vi "LakeShore 336 Curve Manager.vi"() -> ()   [LabVIEW 2021]
doc: "VI to manage calibration curves in Lakeshore model 370 AC resistance Bridge. It will upload, download and display or delete curves. It will always delete a curve before uploading so the input setup may have to be reset after an upload.\nScott Hannahs, <sth@magnet.fsu.edu> NHMFL-FSU, May 2003"
uses:
  Misc Extras/Manufacturer Drivers/LakeShore/Lake Shore Cryotronics 336/Public/Utility/Data Format.ctl
  Sub Controls/ThermListIndex.ctl
  Misc Extras/Manufacturer Drivers/LakeShore/Lake Shore Cryotronics 336/Lake Shore 336.lvlib
panel:
  in  "Done2":bool
  out "XY Graph":cluster{dbl[], dbl[]}(graph)
  out "Curve #":u32[](array[numeric])
  in  "ThermListIndex":T1 max=40 step=20
  in  "stop":bool
  in  "Replace":bool[](array[boolean])=[FALSE, FALSE, FALSE, FALSE, FALSE, FALSE, FALSE, FALSE, FALSE, FALSE, FALSE, FALSE, FALSE, FALSE, FALSE, FALSE, FALSE, FALSE, FALSE, FALSE]
  in  "View":bool[](array[boolean])=[FALSE, FALSE, FALSE, FALSE, FALSE, FALSE, FALSE, FALSE, FALSE, FALSE, FALSE, FALSE, FALSE, FALSE, FALSE, FALSE, FALSE, FALSE, FALSE, FALSE]
  in  "Delete":bool[](array[boolean])=[FALSE, FALSE, FALSE, FALSE, FALSE, FALSE, FALSE, FALSE, FALSE, FALSE, FALSE, FALSE, FALSE, FALSE, FALSE, FALSE, FALSE, FALSE, FALSE, FALSE]
  out "Thermometer List":T3(array[cluster]) {"Temp. Coef" items=["????", "Negative", "Positive"]; "Setpoint Limit" format="%.4f"; "Data Format" items=["mV/K"=1, "V/K"=2, "Ω/K"=3, "Log Ω/K"=4]}
  in  "VISA session":refnum<visa-resource-name>
  out "Model":string="LakeShore Model 370"
  out "Info":string="S/N #000000, Software Date: 20030622"
  # "Name"
  # "Serial #"
  # "Data Format"
  # "Setpoint Limit"
  # "Temp. Coef"
  # "`"
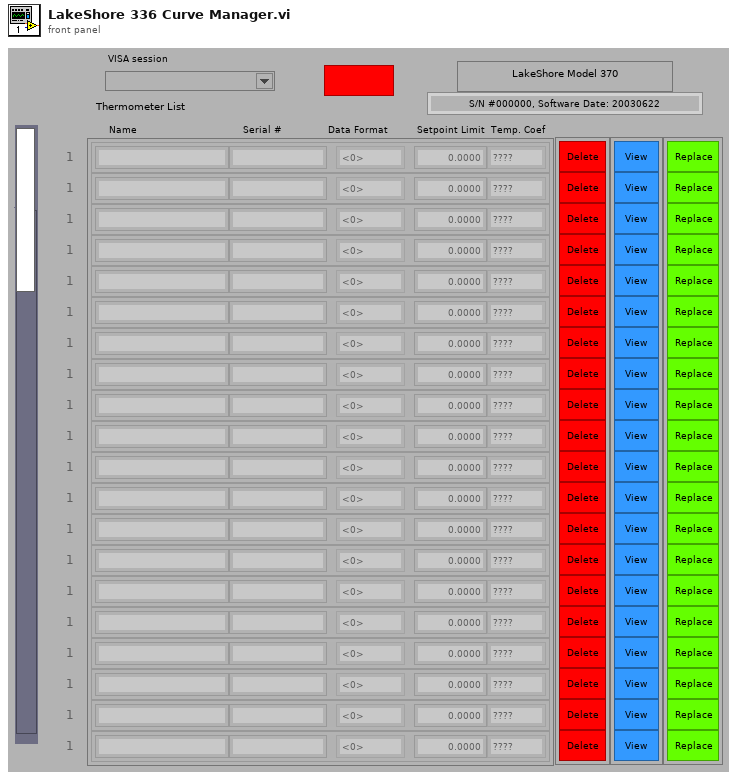
[diagram p1: front panel]
types:
  T1 = typedef "ThermListIndex.ctl" = u32
  T2 = typedef "Data Format.ctl" = u16
  T3 = cluster{"Name":string, "Serial #":string, "Data Format":T2, "Setpoint Limit":dbl, "Temp. Coef":u16}[]
  T4 = cluster{"Curve ID":string, "Serial Number":string, "Data Format":T2, "Setpoint Limit":dbl, "Temp. Coef":u16}[]
  T5 = cluster{"Curve ID":string, "Serial Number":string, "Data Format":T2, "Setpoint Limit":dbl, "Temp. Coef":u16}
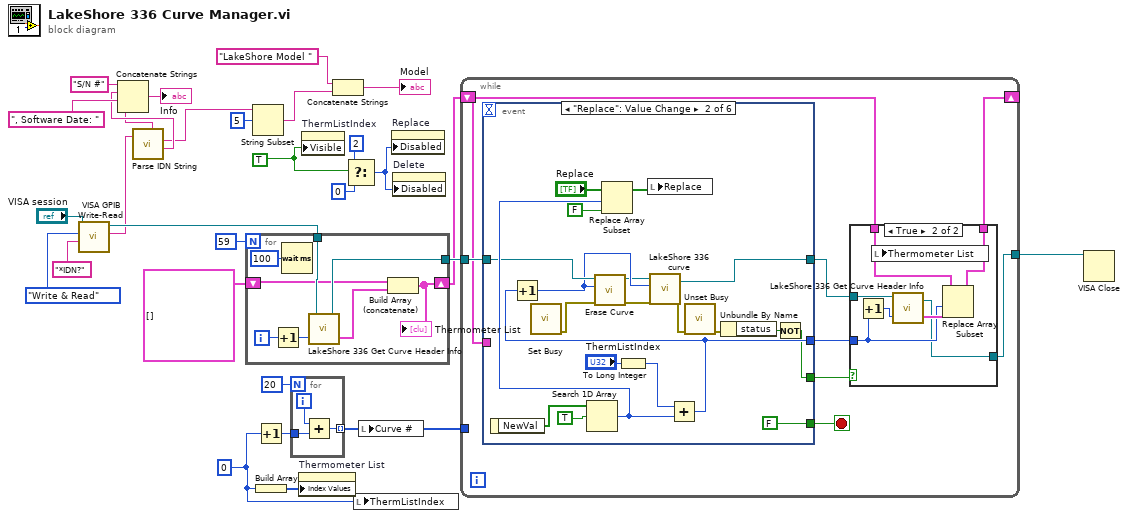
[diagram p0: block diagram]
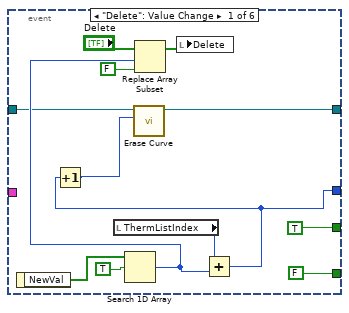
[diagram p3: hidden frame]
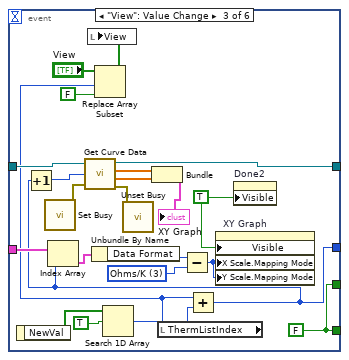
[diagram p4: hidden frame]
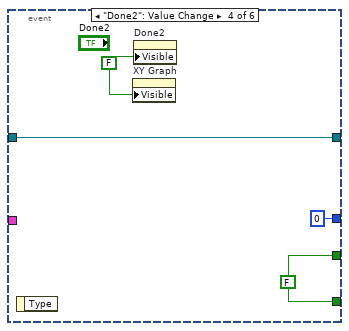
[diagram p5: hidden frame]
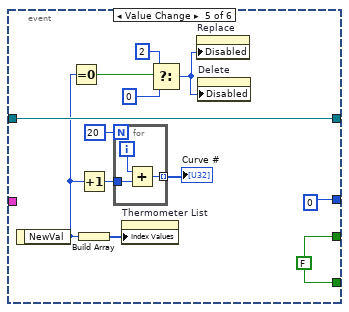
[diagram p6: hidden frame]
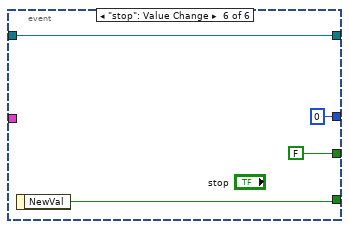
[diagram p7: hidden frame]
diagram:
  w1 = TRUE
  w18 = u32 0
  n1 = call "VISA GPIB Write-Read.vi"("Command"="*IDN?" ("String to Write"), "Action"=enum16{"Write", "Read", "Write & Read"}."Write & Read", "VISA resource name"="VISA session") -> ("String Returned"=w9:string, "dup VISA Session"=w23:refnum<visa-resource-name>)  [unwired: 5 in, 2 out]
  n2 = call "Parse IDN String.vi"("IDN String"=w9) -> ("Info"=w8:string, "Model"=w4:string, "Revision"=w7:string)  [unwired: 1 in, 2 out]
  n3 = Concatenate Strings("S/N #" ("string"), w8, ", Software Date: " ("string"), w7) -> (→"Info":string)
  n4 = for {
    N: 59 -> [_]
    tunnel: w23 -> [w37]
    shift-right: [w32] -> w28
    shift-left: T4 [] -> [w31]
    tunnel: [w33] -> w29
    i -> [w36]
    n5 = Increment(x=w36) -> (x+1=w35:i32)
    n6 = Wait (ms)(milliseconds to wait=u32 100) -> ()  [unwired: 1 out]
    n7 = call "LakeShore 336 Get Curve Header Info.vi"("Curve #"=w35, "VISA session"=w37) -> ("Cluster"=w34:T5, "dup VISA session"=w33:refnum<visa-resource-name>)
    n8 = Build Array (concatenate)(w31, w34) -> (w32:T4)
    "Thermometer List" <- w32
  }
  n9 = String Subset(string=w4, offset (0)=5) -> (substring=w6:string)  [unwired: 1 in]
  n10 = Increment(x=w18) -> (x+1=w21:u32)
  n11 = Build Array(w18) -> (w20:u32[])
  n12 = for {
    N: 20 -> [_]
    tunnel: w21 -> [w40]
    tunnel: [w38] -> w19 mode=indexing
    i -> [w39]
    n13 = Add(x=w39, y=w40) -> (x+y=w38:u32)
  }
  n14 = property on="Thermometer List" class="Arr (strict)"("Index Values"=w20) -> ()  [unwired: 2 in, 2 out]
  n15 = property on="ThermListIndex" class="Slide (strict)"("Visible"=w1) -> ()  [unwired: 2 in, 2 out]
  n16 = Concatenate Strings("LakeShore Model " ("string"), w6) -> (→"Model":string)
  n17 = Select(t=u8 2, s=w1, f=u8 0) -> (s? t:f=w17:u8)
  n18 = local write "ThermListIndex"(w18) -> ()
  n19 = local write "Curve #"(w19) -> ()
  n20 = property on="Replace" class="Arr"("Disabled"=w17) -> ()  [unwired: 2 in, 2 out]
  n21 = property on="Delete" class="Arr"("Disabled"=w17) -> ()  [unwired: 2 in, 2 out]
  n22 = while {
    tunnel: w29 -> [w48]
    shift-right: [w43] -> _
    shift-left: w28 -> [w44]
    tunnel: [w42] -> w2
    tunnel: w19 -> [_]
    stop <- w45 stop-if-true
    n23 = event shown="[1] \"Replace\": Value Change" {
      selector: _ -> [_ _ _ _ _ _]
      dyn-events: _ -> [_ _ _ _ _ _]
      timeout: _ -> [_ _ _ _ _ _]
      tunnel: w48 -> [w59 w74 w111 w114 w129 w134]
      tunnel: [TRUE ("NewVal") w76 w108 w116 w127 FALSE] -> w41
      tunnel: [w61 w81 w93 0 ("index of element") 0 ("index of element") 0 ("index of element")] -> w47
      tunnel: [w58 w88 w110 w114 w129 w134] -> w46
      tunnel: [FALSE ("NewVal") FALSE ("NewVal") w108 w116 w127 w136] -> w45
      tunnel: w44 -> [_ _ w109 _ _ _]
      event "Delete": Value Change {
        n24 = event-data() -> ("NewVal"=w70:bool[])  [unwired: 1 in]
        n25 = local read "ThermListIndex"() -> (w63:T1)
        n26 = Search 1D Array(1D array=w70, element=TRUE) -> (index of element=w62:i32)  [unwired: 1 in]
        n27 = Replace Array Subset(array="Delete", new element=FALSE ("new element/subarray"), index=w62) -> (w65:bool[])
        n28 = local write "Delete"(w65) -> ()
        n29 = Add(x=w63, y=w62) -> (x+y=w61:T1)
        n30 = Increment(x=w61) -> (x+1=w60:T1)
        n31 = call "Erase Curve.vi"("Curve to Erase (21)"=w60, "VISA resource name"=w59) -> ("VISA resource name out"=w58:refnum<visa-resource-name>)  [unwired: 8 in, 1 out]
      }
      event "Replace": Value Change {
        n32 = event-data() -> ("NewVal"=w89:bool[])  [unwired: 1 in]
        n33 = call <vilib>:"Set Busy.vi"() -> ("error out"=w75:errorcluster)  [unwired: 10 in, 1 out]
        n34 = Search 1D Array(1D array=w89, element=TRUE) -> (index of element=w82:i32)  [unwired: 1 in]
        n35 = Replace Array Subset(array="Replace", new element=FALSE ("new element/subarray"), index=w82) -> (w85:bool[])
        n36 = To Long Integer(number="ThermListIndex") -> (32bit integer=w80:i32)
        n37 = local write "Replace"(w85) -> ()
        n38 = Add(x=w80, y=w82) -> (x+y=w81:i32)
        n39 = Increment(x=w81) -> (x+1=w73:i32)
        n40 = call "Erase Curve.vi"("error in (no error)"=w75, "Curve to Erase (21)"=w73, "VISA resource name"=w74) -> ("error out"=w71:errorcluster, "VISA resource name out"=w72:refnum<visa-resource-name>)  [unwired: 7 in]
        n41 = call "LakeShore 336 curve.vi"("error in (no error)"=w71, "Curve"=w73, "VISA session"=w72) -> ("error out"=w79:errorcluster, "dup VISA session"=w88:refnum<visa-resource-name>)  [unwired: 1 in]
        n42 = call <vilib>:"Unset Busy.vi"("error in (no error)"=w79) -> ("error out"=w78:errorcluster)  [unwired: 10 in]
        n43 = Unbundle By Name(w78) -> ("status"=w77:bool)
        n44 = Not(x=w77) -> (.not. x?=w76:bool)
      }
      event "View": Value Change {
        w100 = T2 3 items=["Undefined", "mV/K", "V/K", "Ohms/K", "Log Ohms/K"] ("y")
        w103 = TRUE ("Visible")
        w108 = FALSE ("NewVal")
        n45 = event-data() -> ("NewVal"=w112:bool[])  [unwired: 1 in]
        n46 = call <vilib>:"Set Busy.vi"() -> ("error out"=w92:errorcluster)  [unwired: 10 in, 1 out]
        n47 = Search 1D Array(1D array=w112, element=TRUE) -> (index of element=w94:i32)  [unwired: 1 in]
        n48 = Replace Array Subset(array="View", new element=FALSE ("new element/subarray"), index=w94) -> (w96:bool[])
        n49 = local write "View"(w96) -> ()
        n50 = local read "ThermListIndex"() -> (w95:T1)
        n51 = Add(x=w94, y=w95) -> (x+y=w93:T1)
        n52 = Increment(x=w93) -> (x+1=w107:T1)
        n53 = Index Array(array=w109, index=w93) -> (element=w102:T5)
        n54 = call "Get Curve Data.vi"("VISA session"=w111, "Curve #"=w107, "error in (no error)"=w92) -> ("dup VISA session"=w110:refnum<visa-resource-name>, "Temperature"=w105:dbl[], "Resistance"=w106:dbl[], "error out"=w91:errorcluster)
        n55 = Unbundle By Name(w102) -> ("Data Format"=w101:T2)
        n56 = call <vilib>:"Unset Busy.vi"("error in (no error)"=w91) -> ()  [unwired: 10 in, 1 out]
        n57 = Bundle("Temperature"=w105, "Resistance"=w106) -> (→"XY Graph":cluster{"Temperature":dbl[], "Resistance":dbl[]})  [unwired: 1 in]
        n58 = Subtract(x=w101, y=w100) -> (x-y=w99:T2)
        n59 = property on="XY Graph" class="XYGraph (strict)"("Visible"=w103, "X Scale.Mapping Mode"=w99, "Y Scale.Mapping Mode"=w99) -> ()  [unwired: 2 in, 2 out]
        n60 = property on="Done2" class="Bool"("Visible"=w103) -> ()  [unwired: 2 in, 2 out]
      }
      event "Done2": Value Change {
        w116 = FALSE
        w117 = FALSE ("Visible")
        n61 = event-data() -> ()  [unwired: 1 in, 1 out]
        n62 = property on="XY Graph" class="XYGraph (strict)"("Visible"=w117) -> ()  [unwired: 2 in, 2 out]
        n63 = property on="Done2" class="Bool"("Visible"=w117) -> ()  [unwired: 2 in, 2 out]
      }
      event Value Change {
        w127 = FALSE
        n64 = event-data() -> ("NewVal"=w122:T1)  [unwired: 1 in]
        n65 = Equal To 0?(x=w122) -> (x = 0?=w118:bool)
        n66 = Increment(x=w122) -> (x+1=w125:T1)
        n67 = Build Array(w122) -> (w126:T1[])
        n68 = for {
          N: 20 -> [_]
          tunnel: w125 -> [w132]
          tunnel: [w130] -> w124 mode=indexing
          i -> [w131]
          n69 = Add(x=w131, y=w132) -> (x+y=w130:T1)
        }
        "Curve #" <- w124
        n70 = property on="Thermometer List" class="Arr (strict)"("Index Values"=w126) -> ()  [unwired: 2 in, 2 out]
        n71 = Select(t=u8 2, s=w118, f=u8 0) -> (s? t:f=w119:u8)
        n72 = property on="Replace" class="Arr"("Disabled"=w119) -> ()  [unwired: 2 in, 2 out]
        n73 = property on="Delete" class="Arr"("Disabled"=w119) -> ()  [unwired: 2 in, 2 out]
      }
      event "stop": Value Change {
        n74 = event-data() -> ("NewVal"=w136:bool)  [unwired: 1 in]
      }
    }
    n75 = case shown="True" w41 {
      tunnel: w47 -> [_ w55]
      tunnel: w46 -> [w49 w54]
      tunnel: w44 -> [w50 w53]
      tunnel: [w50 w51] -> w43
      tunnel: [w49 w52] -> w42
      frame False {
      }
      frame True {
        n76 = Increment(x=w55) -> (x+1=w56:T1)
        n77 = call "LakeShore 336 Get Curve Header Info.vi"("Curve #"=w56, "VISA session"=w54) -> ("Cluster"=w57:T5, "dup VISA session"=w52:refnum<visa-resource-name>)
        n78 = Replace Array Subset(array=w53, new element=w57, index=w55) -> (w51:T4)
        n79 = local write "Thermometer List"(w51) -> ()
      }
    }
  }
  n80 = VISA Close(VISA resource name=w2) -> ()  [unwired: 1 in, 1 out]
